vi "WeightUpdate.vi"(9 "(dE/dOut)(PrevLayerOP)":dbl[](array[numeric]), 10 "Learning Rate":dbl, 11 "weights":dbl[](array[numeric])) -> (2 "dE/dWi":dbl[](array[numeric]), 3 "w+":dbl[](array[numeric]))   [LabVIEW 2014]
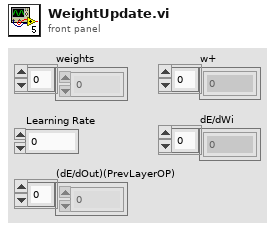
[diagram p1: front panel]
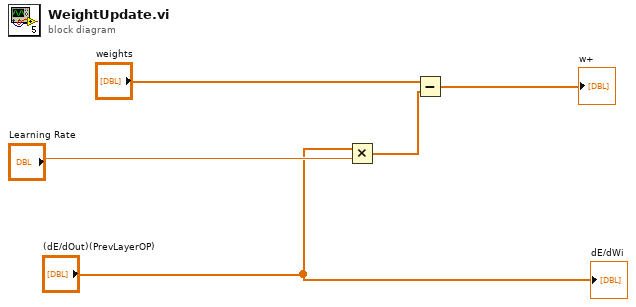
[diagram p0: block diagram]
diagram:
  n1 = Multiply(x="(dE/dOut)(PrevLayerOP)", y="Learning Rate") -> (x*y=w3:dbl[])
  n2 = Subtract(x="weights", y=w3) -> (x-y=→"w+":dbl[])
  "dE/dWi" <- "(dE/dOut)(PrevLayerOP)"
